vi "PCA Compute.vi"   [LabVIEW 2020, in "OpenLvVision_OpenCv.lvlib" / "PCA.lvclass"]
doc: "Performs PCA of the supplied dataset. It is safe to reuse the same PCA structure for multiple datasets. That is, if the structure has been previously used with another dataset, the existing internal data is reclaimed and the new eigenvalues, eigenvectors and mean are allocated and computed."
uses:
  PCA.lvclass
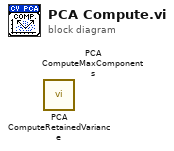
[diagram p0: block diagram]
diagram:
  n1 = call "PCA ComputeRetainedVariance.vi"() -> ()  [unwired: 10 in, 2 out]
  n2 = call "PCA ComputeMaxComponents.vi"() -> ()  [unwired: 10 in, 2 out]
